vi "CPU Info.Query Core Count.vi"(8 "error in (no error)":errorcluster, 11 "CPU Info in":refnum<class "CPU Info.lvclass">) -> (0 "error out":errorcluster, 2 "Core Count":i32, 3 "CPU Info out":refnum<class "CPU Info.lvclass">)   [LabVIEW 2017, in "DSF Core.lvlib" / "CPU Info.lvclass"]
uses:
  CPU Info.lvclass
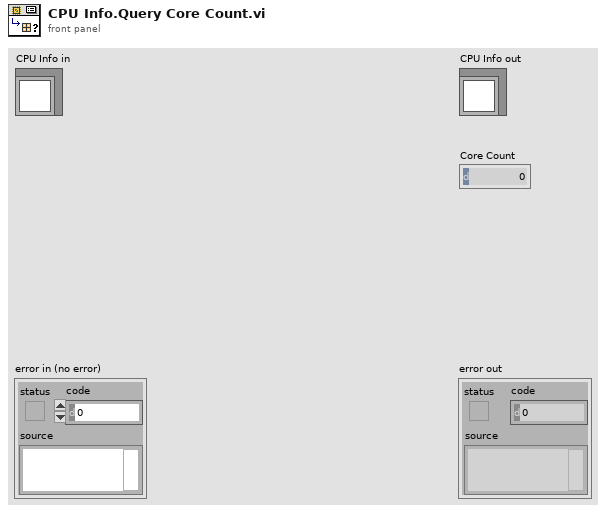
[diagram p1: front panel]
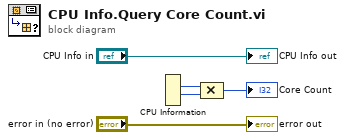
[diagram p0: block diagram]
diagram:
  n1 = CPU Information() -> (5:w2:i32, 6:w3:i32)  [unwired: 2 out]
  n2 = Compound Arithmetic op=MULTIPLY(w2, w3) -> (→"Core Count":i32)
  "error out" <- "error in (no error)"
  "CPU Info out" <- "CPU Info in"
